vi "write_params.vi"(8 "error in (no error)":errorcluster, 10 "params":T1={"alpha"={"alpha_type"="float", "alpha_float"=1.0, "alpha_list"=[]}, "kernel"="linear", "gamma"={"gamma_type"="None", "gamma_float"=0.0}, "degree"=3.0, "coef0"=1.0}, 11 "KernelRidge in":refnum<class "KernelRidge.lvclass">) -> (0 "error out":errorcluster, 3 "KernelRidge out":refnum<class "KernelRidge.lvclass">)   [LabVIEW 2020, in "KernelRidge.lvclass"]
uses:
  KernelRidge.lvclass
  Controls/kernel_ridge_params.ctl
  KernelRidge.lvclass/KernelRidge.ctl
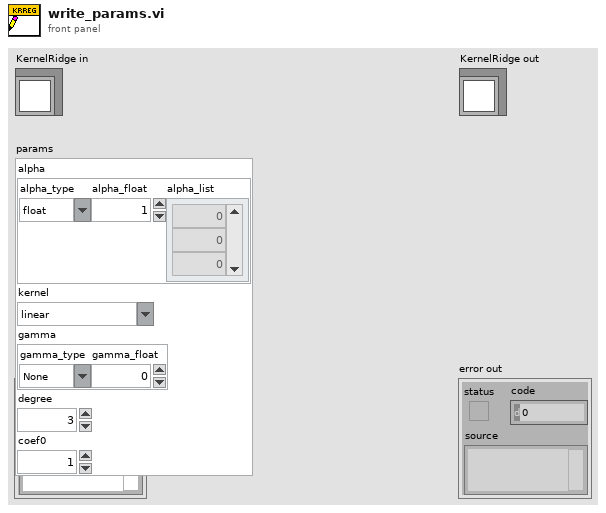
[diagram p1: front panel]
types:
  T1 = typedef "kernel_ridge_params.ctl" = cluster{"alpha":cluster{"alpha_type":string, "alpha_float":dbl, "alpha_list":dbl[]}, "kernel":string, "gamma":cluster{"gamma_type":string, "gamma_float":dbl}, "degree":dbl, "coef0":dbl}
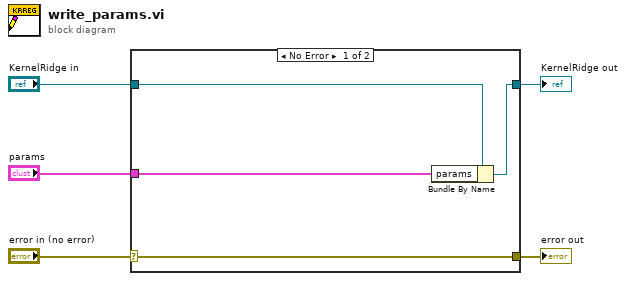
[diagram p0: block diagram]
diagram:
  n1 = case shown="No Error" "error in (no error)" {
    selector: "error in (no error)" -> [w9 w10]
    tunnel: [w9 w10] -> w4
    tunnel: [w7 w11] -> w2
    tunnel: "KernelRidge in" -> [w8 w11]
    tunnel: "params" -> [w6 _]
    frame No Error {
      n2 = Bundle By Name(cluster=w8, "params"=w6) -> (w7:refnum<class "KernelRidge.lvclass">)
    }
    frame Error {
    }
  }
  "error out" <- w4
  "KernelRidge out" <- w2
